vi "Initialize.vi"(7 "Serial Configuration":T1={"Baud Rate"=115200, "Parity"=enum."None", "Data Bits"=8, "Stop Bits"=10, "Flow Control"=0} {"Flow Control" items=["None", "XON/XOFF", "RTS/CTS", "XON/XOFF & RTS/CTS", "DTR/DSR", "XON/XOFF & DTR/DSR"]; "Stop Bits" items=["1.0"=10, "1.5"=15, "2.0"=20]; "Data Bits" items=["7"=7, "8"=8]; "Baud Rate" items=["300"=300, "600"=600, "1200"=1200, "2400"=2400, "4800"=4800, "9600"=9600, "19200"=19200, "38400"=38400, "57600"=57600, "115200"=115200]}, 8 "error in (no error)":errorcluster, 11 "VISA resource name":refnum<visa-resource-name>) -> (0 "error out":errorcluster, 3 "VISA resource name out":refnum<visa-resource-name>)   [LabVIEW 2020, in "CAEN PSM.lvlib"]
doc: "Establishes communication with the instrument. Therefore, call this VI before calling other instrument driver VIs for this instrument. Generally, you need to call the Initialize VI only once at the beginning of an application."
uses:
  CAEN PSM.lvlib
  VISA Open Access Mode.ctl
  Select Event Type.ctl
panel:
  # "(c) 2012 CAEN SpA.  ALL RIGHTS RESERVED."
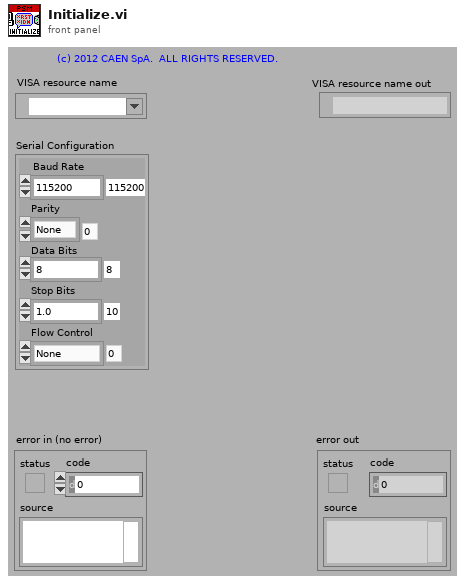
[diagram p1: front panel]
types:
  T1 = cluster{"Baud Rate":u32, "Parity":enum16{"None", "Odd", "Even", "Mark", "Space"}, "Data Bits":u16, "Stop Bits":u16, "Flow Control":u16}
  T2 = typedef "VISA Open Access Mode.ctl" = u32
  T3 = typedef "Select Event Type.ctl" = u32
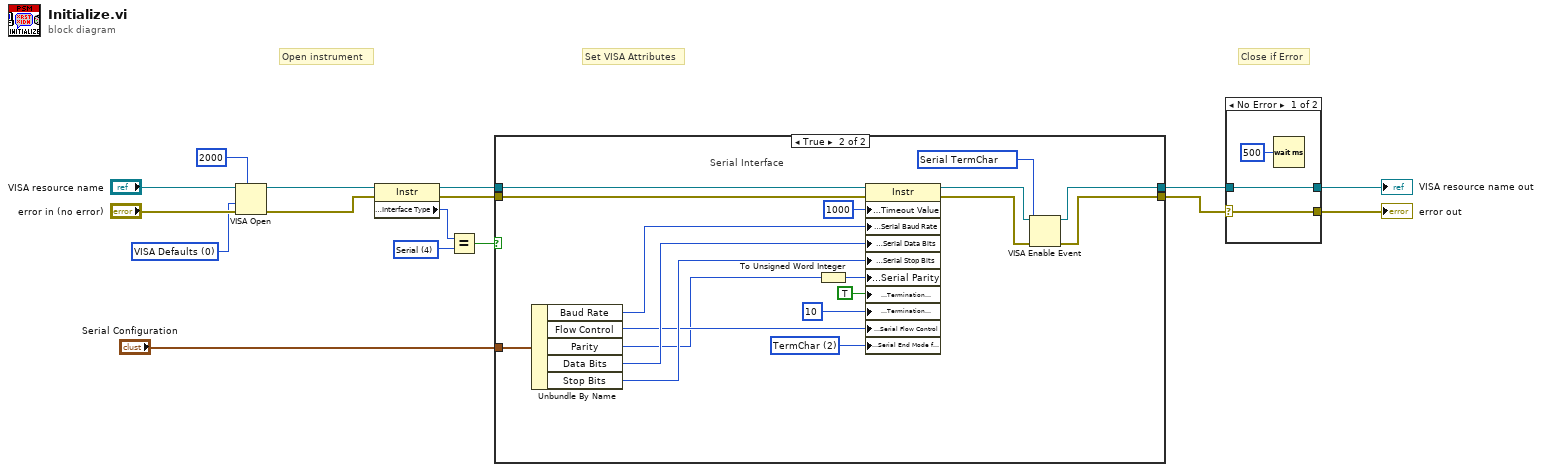
[diagram p0: block diagram]
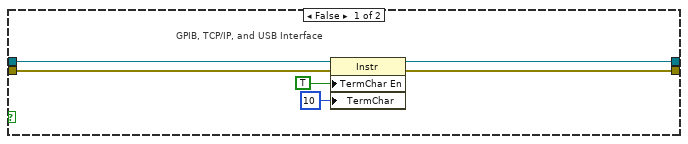
[diagram p2: hidden frame]
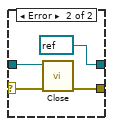
[diagram p3: hidden frame]
diagram:
  w2 = T2 0 items=["VISA Defaults"=0, "Exclusive Lock"=1, "Load Configured Settings"=4] ("Access Mode")
  w10 = u16 4 items=["GPIB"=1, "VXI"=2, "GPIB-VXI"=3, "Serial"=4, "PXI"=5, "TCPIP"=6, "USB"=7] ("Interface Information:Interface Type")
  # "Set VISA Attributes"
  # "Close if Error"
  # "Open instrument"
  n1 = VISA Open(timeout (0)=u32 2000 ("VISA Open timeout (0)"), access mode=w2, error in (no error)="error in (no error)", VISA resource name="VISA resource name") -> (VISA resource name=w5:refnum<visa-resource-name>, error out=w4:errorcluster)  [unwired: 1 in]
  n2 = property class="Instr"(reference=w5, error in=w4) -> (reference out=w13:refnum<visa-resource-name>, error out=w12:errorcluster, "Interface Information:Interface Type"=w14:u16)
  n3 = Equal?(x=w14, y=w10) -> (x = y?=w11:bool)
  n4 = case shown="True" w11 {
    tunnel: [w19 w24] -> w7
    tunnel: [w20 w25] -> w6
    tunnel: w13 -> [w22 w39]
    tunnel: w12 -> [w21 w38]
    tunnel: "Serial Configuration" -> [_ w40]
    frame False {
      # "GPIB, TCP/IP, and USB Interface"
      n5 = property class="Instr"(reference=w22, error in=w21, "TermChar En"=TRUE ("Message Based Settings:Termination Character Enable"), "TermChar"=u8 10 ("Message Based Settings:Termination Character")) -> (reference out=w19:refnum<visa-resource-name>, error out=w20:errorcluster)
    }
    frame True {
      w23 = T3 1073684516 items=["Service Request"=1073684491, "Trigger"=3221168138, "Clear"=1073684493, "VXI Signal"=1073684512, "VXI/VME Interrupt"=3221168161, "VXI/VME Sysfail"=1073684509, "VXI/VME Sysreset"=1073684510, "GPIB CIC"=1073684498, "GPIB Talk"=1073684499, "GPIB Listen"=1073684500, "PXI Interrupt"=1073684514, "Serial Break"=1073684515, "Serial TermChar"=1073684516, "Serial CTS"=1073684521, "Serial DSR"=1073684522, "Serial DCD"=1073684524, "Serial RI"=1073684526, "Serial Character"=1073684533, "USB Interrupt"=1073684535, "All Enabled"=1073709055] ("Event Type")
      w28 = u16 2 items=["None", "Last Bit", "TermChar"] ("Serial Settings:End Mode for Reads")
      # "Serial Interface"
      n6 = Unbundle By Name(w40) -> ("Baud Rate"=w37:u32, "Flow Control"=w34:u16, "Parity"=w33:enum16{"None", "Odd", "Even", "Mark", "Space"}, "Data Bits"=w36:u16, "Stop Bits"=w35:u16)
      n7 = To Unsigned Word Integer(number=w33) -> (unsigned 16bit integer=w32:u16)
      n8 = property class="Instr"(reference=w39, error in=w38, "General Settings:Timeout Value"=u32 1000, "Serial Settings:Serial Baud Rate"=w37, "Serial Settings:Serial Data Bits"=w36, "Serial Settings:Serial Stop Bits"=w35, "Serial Settings:Serial Parity"=w32, "Message Based Settings:Termination Character Enable"=TRUE, "Message Based Settings:Termination Character"=u8 10, "Serial Settings:Serial Flow Control"=w34, "Serial Settings:Serial End Mode for Reads"=w28) -> (reference out=w27:refnum<visa-resource-name>, error out=w26:errorcluster)
      n9 = VISA Enable Event(8:w26, 10:w23, 11:w27) -> (0:w25:errorcluster, 3:w24:refnum<visa-resource-name>)  [unwired: 1 in]
    }
  }
  n10 = case shown="No Error" w6 {
    selector: w6 -> [w42 w45]
    tunnel: w7 -> [w43 w46]
    tunnel: [w43 refnum<visa-resource-name> refnum ("VISA resource name out")] -> w9
    tunnel: [w42 w47] -> w8
    frame No Error {
      n11 = Wait (ms)(milliseconds to wait=u32 500) -> ()  [unwired: 1 out]
    }
    frame Error {
      n12 = call "Close.vi"("error in (no error)"=w45, "VISA resource name"=w46) -> ("error out"=w47:errorcluster)  [unwired: 9 in]
    }
  }
  "VISA resource name out" <- w9
  "error out" <- w8
